vi "Playback Frame Cropping.vi"(8 "error in (no error)":errorcluster, 11 "Frame Grabber Data in":T2={"Camera Session"="", "Frame"=refnum, "AVI Refnum"=refnum, "Codecs"=[], "Frame number"=0, "Tracking File Refnum"=refnum, "Tick Count"=0, "Probe Object"=refnum, "Playback Probe Data"=[], "Rigid Body"={"Position"={"x (mm)"=0.0, "y (mm)"=0.0, "z (mm)"=0.0}, "Orientation"={"Pitch (rad)"=0.0, "Yaw (rad)"=0.0, "Roll (rad)"=0.0}, "Quaternion"={"qx"=0.0, "qy"=0.0, "qz"=0.0, "qw"=0.0}, "Tracked?"=FALSE}, "Total no frames playback"=0, "Video FPS"=0.0, "Camera connected?"=FALSE, "Scene"=refnum, "Cropped Frame"=refnum, "Tracker FPS"=0.0, "Crop ROI"=[], "Presentation Values"=[], "Elapsed time (ms)"=0, "Camera frames playback"=0, "Refnums"={"Live Refnum"=refnum, "Record Refnum"=refnum, "Recording Settings Refnum"=refnum, "Playback Refnum"=refnum, "Frame Slider Refnum"=refnum, "Pause Refnum"=refnum, "Home Refnum"=refnum, "Crop Refnum"=refnum, "Clear Crop Refnum"=refnum, "stop refnum"=refnum, "Playback Rate Refnum"=refnum, "Operator Settings Refnums"=refnum, "Presentation Refnum"=refnum, "Gestation Refnum"=refnum, "Crop Time Frame Slider Refnum"=refnum, "Cancel Save Refnum"=refnum, "Reverse Playback Refnum"=refnum, "Connection Settings Refnum"=refnum}, "Dimensions"={"Probe Dimensions"={"Probe Width"=0.0, "Probe Depth"=1.0, "Probe Height"=0.0}, "Room Dimensions"={"Room Width"=0.0, "Room Depth"=0.0, "Room Height"=0.0}}, "Playback Data As Strings"=[], "Cropped Tracking File Refnum"=refnum, "Cropped AVI Refnum"=refnum, "Header"=[], "Total euclidian distance"=0.0, "Annotation File Path"=path "", "Playback File Path"=path ""}) -> (0 "error out":errorcluster, 1 "Continue playback?":bool, 2 "Image":T1, 3 "Frame Grabber Data out":T2={"Camera Session"="", "Frame"=refnum, "AVI Refnum"=refnum, "Codecs"=[], "Frame number"=0, "Tracking File Refnum"=refnum, "Tick Count"=0, "Probe Object"=refnum, "Playback Probe Data"=[], "Rigid Body"={"Position"={"x (mm)"=0.0, "y (mm)"=0.0, "z (mm)"=0.0}, "Orientation"={"Pitch (rad)"=0.0, "Yaw (rad)"=0.0, "Roll (rad)"=0.0}, "Quaternion"={"qx"=0.0, "qy"=0.0, "qz"=0.0, "qw"=0.0}, "Tracked?"=FALSE}, "Total no frames playback"=0, "Video FPS"=0.0, "Camera connected?"=FALSE, "Scene"=refnum, "Cropped Frame"=refnum, "Tracker FPS"=0.0, "Crop ROI"=[], "Presentation Values"=[], "Elapsed time (ms)"=0, "Camera frames playback"=0, "Refnums"={"Live Refnum"=refnum, "Record Refnum"=refnum, "Recording Settings Refnum"=refnum, "Playback Refnum"=refnum, "Frame Slider Refnum"=refnum, "Pause Refnum"=refnum, "Home Refnum"=refnum, "Crop Refnum"=refnum, "Clear Crop Refnum"=refnum, "stop refnum"=refnum, "Playback Rate Refnum"=refnum, "Operator Settings Refnums"=refnum, "Presentation Refnum"=refnum, "Gestation Refnum"=refnum, "Crop Time Frame Slider Refnum"=refnum, "Cancel Save Refnum"=refnum, "Reverse Playback Refnum"=refnum, "Connection Settings Refnum"=refnum}, "Dimensions"={"Probe Dimensions"={"Probe Width"=0.0, "Probe Depth"=1.0, "Probe Height"=0.0}, "Room Dimensions"={"Room Width"=0.0, "Room Depth"=0.0, "Room Height"=0.0}}, "Playback Data As Strings"=[], "Cropped Tracking File Refnum"=refnum, "Cropped AVI Refnum"=refnum, "Header"=[], "Total euclidian distance"=0.0, "Annotation File Path"=path "", "Playback File Path"=path ""}, 4 "Time elapsed (s)":dbl, 5 "Camera frame number":u32)   [LabVIEW 2017]
uses:
  Controls/Frame Grabber Data.ctl
  <vilib>/userdefined/High Color/IMAQdx.ctl
  <vilib>/vision/Image Controls.llb/IMAQ Image.ctl
  <vilib>/vision/Avi.llb/IMAQ AVI2 Refnum.ctl
  Controls/Rigid Body Info.ctl
  Controls/Position.ctl
  Controls/Orientation.ctl
  Controls/Refnums.ctl
  Controls/Recording Settings.ctl
  Controls/Operator Settings.ctl
  Controls/Operator.ctl
  Controls/Connection Settings.ctl
  Controls/Tracker Type.ctl
  Controls/COM Port.ctl
  Controls/Dimensions.ctl
  Controls/Room Dimensions.ctl
  <vilib>/vision/NI_Vision_Development_Module.lvlib
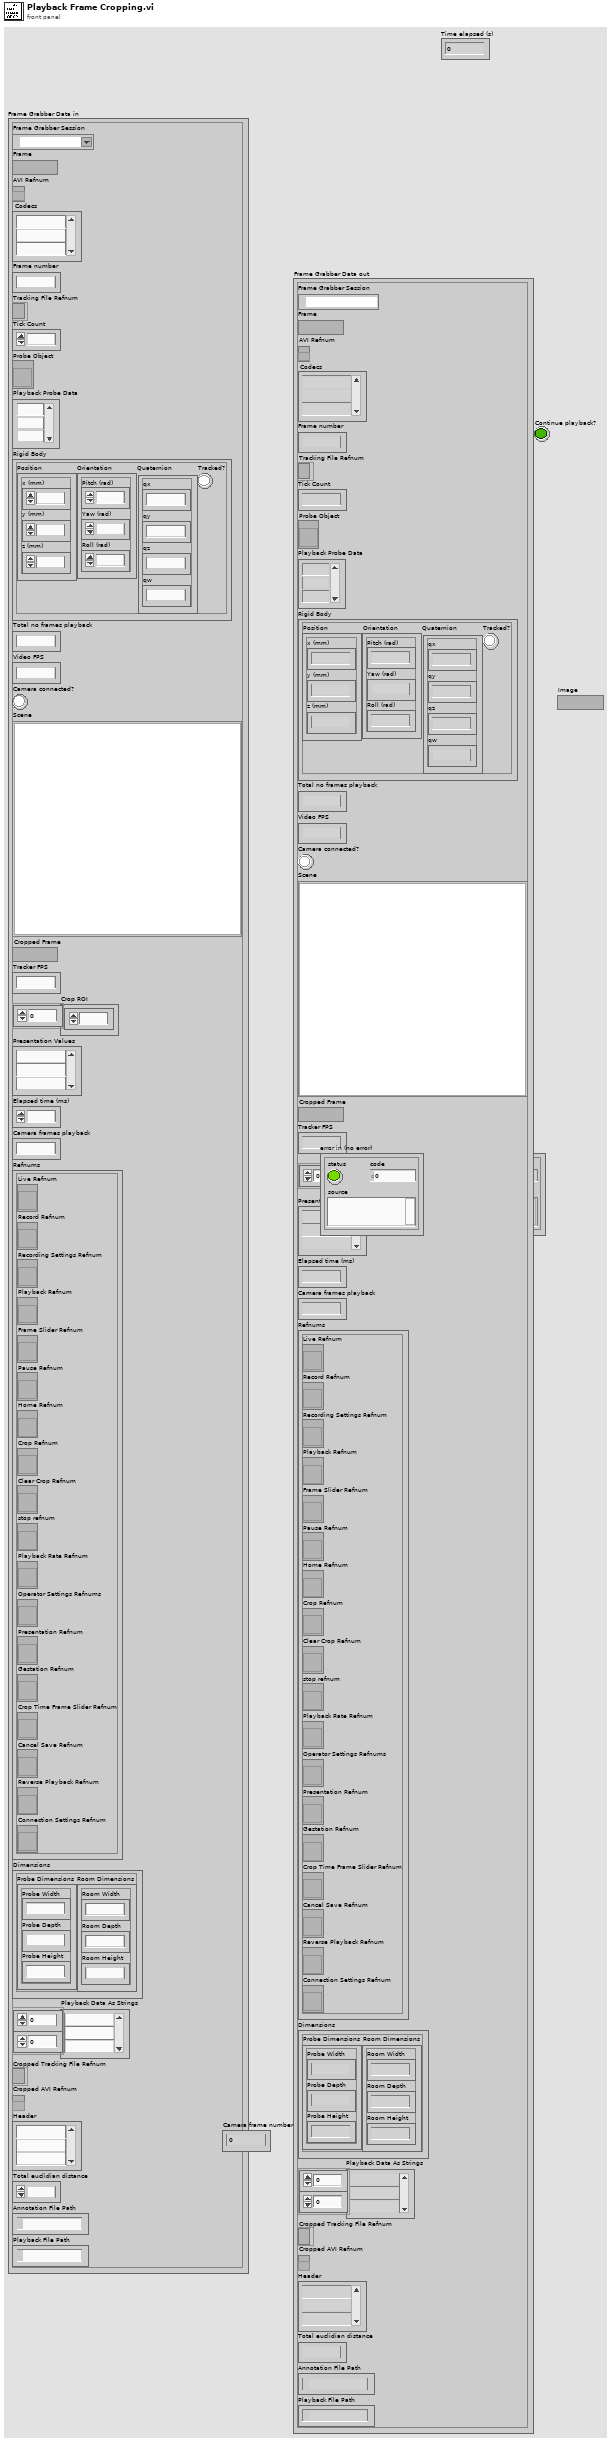
[diagram p1: front panel]
types:
  T1 = typedef "IMAQ Image.ctl" = refnum<image>
  T2 = typedef "Frame Grabber Data.ctl" = cluster{"Camera Session":T3, "Frame":T1, "AVI Refnum":T4, "Codecs":string[], "Frame number":u32, "Tracking File Refnum":refnum<file>, "Tick Count":u32, "Probe Object":refnum<vi>, "Playback Probe Data":dbl[][], "Rigid Body":T5, "Total no frames playback":i32, "Video FPS":dbl, "Camera connected?":bool, "Scene":refnum<vi>, "Cropped Frame":T1, "Tracker FPS":dbl, "Crop ROI":i32[], "Presentation Values":string[], "Elapsed time (ms)":u32, "Camera frames playback":u32, "Refnums":T8, "Dimensions":T9, "Playback Data As Strings":string[][], "Cropped Tracking File Refnum":refnum<file>, "Cropped AVI Refnum":T4, "Header":string[], "Total euclidian distance":dbl, "Annotation File Path":path, "Playback File Path":path}
  T3 = typedef "IMAQdx.ctl" = refnum<k21>
  T4 = typedef "IMAQ AVI2 Refnum.ctl" = refnum<k20>
  T5 = typedef "Rigid Body Info.ctl" = cluster{"Position":T6, "Orientation":T7, "Quaternion":cluster{"qx":sgl, "qy":sgl, "qz":sgl, "qw":sgl}, "Tracked?":bool}
  T6 = typedef "Position.ctl" = cluster{"x (mm)":sgl, "y (mm)":sgl, "z (mm)":sgl}
  T7 = typedef "Orientation.ctl" = cluster{"Pitch (rad)":sgl, "Yaw (rad)":sgl, "Roll (rad)":sgl}
  T8 = typedef "Refnums.ctl" = cluster{"Live Refnum":refnum<vi>, "Record Refnum":refnum<vi>, "Recording Settings Refnum":refnum<vi>, "Playback Refnum":refnum<vi>, "Frame Slider Refnum":refnum<vi>, "Pause Refnum":refnum<vi>, "Home Refnum":refnum<vi>, "Crop Refnum":refnum<vi>, "Clear Crop Refnum":refnum<vi>, "stop refnum":refnum<vi>, "Playback Rate Refnum":refnum<vi>, "Operator Settings Refnums":refnum<vi>, "Presentation Refnum":refnum<vi>, "Gestation Refnum":refnum<vi>, "Crop Time Frame Slider Refnum":refnum<vi>, "Cancel Save Refnum":refnum<vi>, "Reverse Playback Refnum":refnum<vi>, "Connection Settings Refnum":refnum<vi>}
  T9 = typedef "Dimensions.ctl" = cluster{"Probe Dimensions":cluster{"Probe Width":sgl, "Probe Depth":sgl, "Probe Height":sgl}, "Room Dimensions":T10}
  T10 = typedef "Room Dimensions.ctl" = cluster{"Room Width":dbl, "Room Depth":dbl, "Room Height":dbl}
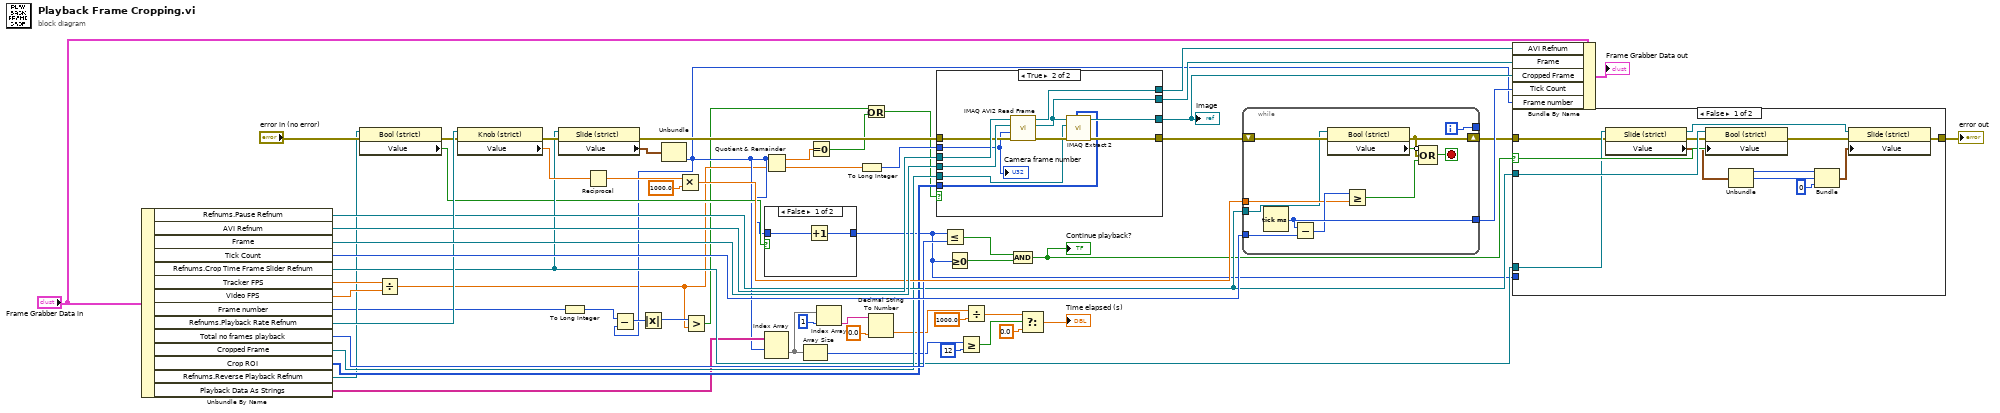
[diagram p0: block diagram]
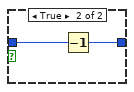
[diagram p2: hidden frame]
diagram:
  n1 = Unbundle By Name("Frame Grabber Data in") -> ("Refnums.Pause Refnum"=w38:refnum<vi>, "AVI Refnum"=w59:T4, "Frame"=w60:T1, "Tick Count"=w53:u32, "Refnums.Crop Time Frame Slider Refnum"=w34:refnum<vi>, "Tracker FPS"=w52:dbl, "Video FPS"=w51:dbl, "Frame number"=w7:u32, "Refnums.Playback Rate Refnum"=w45:refnum<vi>, "Total no frames playback"=w44:i32, "Cropped Frame"=w37:T1, "Crop ROI"=w36:i32[], "Refnums.Reverse Playback Refnum"=w30:refnum<vi>, "Playback Data As Strings"=w25:string[][])
  n2 = property class="Bool (strict)"(reference=w30, error in="error in (no error)") -> (error out=w31:errorcluster, "Value"=w29:bool)  [unwired: 1 out]
  n3 = Divide(x=w52, y=w51) -> (x/y=w3:dbl)
  n4 = property class="Knob (strict)"(reference=w45, error in=w31) -> (error out=w46:errorcluster, "Value"=w47:dbl)  [unwired: 1 out]
  n5 = property class="Slide (strict)"(reference=w34, error in=w46) -> (error out=w49:errorcluster, "Value"=w41:cluster{i32, i32, i32})  [unwired: 1 out]
  n6 = To Long Integer(number=w7) -> (32bit integer=w5:i32)
  n7 = Reciprocal(x=w47) -> (1/x=w56:dbl)
  n8 = Unbundle(w41) -> (w6:i32)  [unwired: 2 out]
  n9 = Subtract(x=w5, y=w6) -> (x-y=w8:i32)
  n10 = Absolute Value(x=w8) -> (abs(x)=w4:i32)
  n11 = Multiply(x=w56, y=1000.0) -> (x*y=w54:dbl)
  n12 = Greater?(x=w4, y=w3) -> (0:w2:bool)
  n13 = case shown="False" w29 {
    tunnel: [w62 w63] -> w27
    tunnel: w6 -> [w61 w64]
    frame False {
      n14 = Increment(x=w61) -> (x+1=w62:i32)
    }
    frame True {
      n15 = Decrement(x=w64) -> (x-1=w63:i32)
    }
  }
  n16 = Index Array(array=w25, index (row)=w6) -> (element=w21:string[])  [unwired: 1 in]
  n17 = Quotient & Remainder(x=w6, y=w3) -> (x-y*floor(x/y)=w10:dbl, floor(x/y)=w50:dbl)
  n18 = Array Size(array=w21) -> (size(s)=w24:i32)
  n19 = Equal To 0?(x=w10) -> (x = 0?=w9:bool)
  n20 = Index Array(array=w21, index=1) -> (element=w19:string)
  n21 = To Long Integer(number=w50) -> (32bit integer=w43:i32)
  n22 = Or(x=w2, y=w9) -> (x .or. y?=w1:bool)
  n23 = Decimal String To Number(string=w19, default (0L)=0.0 ("default (0 I32)")) -> (number=w17:dbl)  [unwired: 1 in, 1 out]
  n24 = case shown="True" w1 {
    tunnel: [w66 w73] -> w12
    tunnel: w60 -> [w67 w79]
    tunnel: w59 -> [w65 w78]
    tunnel: [w68 w74] -> w48
    tunnel: w49 -> [w68 w77]
    tunnel: w43 -> [_ w76]
    tunnel: w37 -> [w66 w70]
    tunnel: w36 -> [_ w72]
    tunnel: [w67 w71] -> w35
    tunnel: [w65 w69] -> w26
    frame False {
    }
    frame True {
      n25 = call "IMAQ AVI2 Read Frame"("error in (no error)"=w77, "Frame Number"=w76, "Image"=w79, "AVI Refnum"=w78) -> ("error out"=w75:errorcluster, "Image Out"=w71:T1, "AVI Refnum (duplicate)"=w69:T4)  [unwired: 5 in]
      n26 = call "IMAQ Extract 2"("Optional Rectangle"=w72, "error in (no error)"=w75, "Image Dst"=w70, "Image Src"=w71) -> ("error out"=w74:errorcluster, "Image Dst Out"=w73:T1)  [unwired: 6 in]
      "Camera frame number" <- w76
    }
  }
  "Image" <- w12
  n27 = Less Or Equal?(x=w27, y=w44) -> (x <= y?=w39:bool)
  n28 = Greater Or Equal To 0?(x=w27) -> (x >= 0?=w28:bool)
  n29 = Greater Or Equal?(x=w24, y=12) -> (x >= y?=w22:bool)
  n30 = Divide(x=w17, y=1000.0) -> (x/y=w15:dbl)
  n31 = And(x=w39, y=w28) -> (x .and. y?=w33:bool)
  "Continue playback?" <- w33
  n32 = Select(t=w15, s=w22, f=0.0) -> (s? t:f=→"Time elapsed (s)":dbl)
  n33 = while {
    tunnel: [w90] -> w57
    tunnel: w54 -> [w88]
    tunnel: w53 -> [w87]
    shift-right: [w83] -> w42
    shift-left: w48 -> [w84]
    tunnel: w38 -> [w82]
    tunnel: [w80] -> _
    i -> [w80]
    stop <- w86 stop-if-true
    n34 = Tick Count (ms)() -> (millisecond timer value=w90:u32)
    n35 = Subtract(x=w90, y=w87) -> (x-y=w89:u32)
    n36 = property class="Bool (strict)"(reference=w82, error in=w84) -> (error out=w83:errorcluster, "Value"=w81:bool)  [unwired: 1 out]
    n37 = Greater Or Equal?(x=w89, y=w88) -> (x >= y?=w85:bool)
    n38 = Compound Arithmetic op=OR(invert w81, w83, w85) -> (w86:bool)
  }
  n39 = Bundle By Name(cluster="Frame Grabber Data in", "AVI Refnum"=w26, "Frame"=w35, "Cropped Frame"=w12, "Tick Count"=w57, "Frame number"=w6) -> (→"Frame Grabber Data out":T2)
  n40 = case shown="False" w33 {
    selector: w33 -> [w101 _]
    tunnel: w42 -> [w99 w104]
    tunnel: w38 -> [w102 _]
    tunnel: w27 -> [_ _]
    tunnel: w34 -> [w100 _]
    tunnel: [w91 w104] -> w11
    frame False {
      n41 = property class="Slide (strict)"(reference=w100, error in=w99) -> (reference out=w94:refnum<vi>, error out=w98:errorcluster, "Value"=w97:cluster{i32, i32, i32})
      n42 = property class="Bool (strict)"(reference=w102, error in=w98, "Value"=w101) -> (error out=w93:errorcluster)  [unwired: 1 out]
      n43 = Unbundle(w97) -> (w95:i32, w96:i32)  [unwired: 1 out]
      n44 = Bundle(w95, w96, u32 0) -> (w92:cluster{i32, i32, u32})  [unwired: 1 in]
      n45 = property class="Slide (strict)"(reference=w94, error in=w93, "Value"=w92) -> (error out=w91:errorcluster)  [unwired: 1 out]
    }
    frame True {
    }
  }
  "error out" <- w11
